vi "Initialize.vi"(8 "error in":errorcluster, 10 "parameters":variant, 11 "node in":refnum<class "control module editor.lvclass">) -> (0 "error out":errorcluster, 2 "summary":T2[](array[typedef]), 3 "data value reference":T1)   [LabVIEW 2013, in "control module editor.lvclass"]
doc: "Initializes the data of a node to its default state.\nThe object is not created inside of this VI, because it is created from a File depending on user selection."
uses:
  control module editor.lvclass
  <vilib>/NI/Configuration Framework/Node/Summary.ctl
  <vilib>/NI/Configuration Framework/Node/NodeRef.ctl
  <vilib>/NI/Configuration Framework/Node/NISE_CEF_Node.lvclass
  Configuration Editor/Classes/Module editor node/module editor node.lvclass
  configuration/control module configuration.lvclass
  read fixed channel configuration.vi
  <vilib>/NI/Configuration Framework/NISE_CEF_TreeControl.lvlib
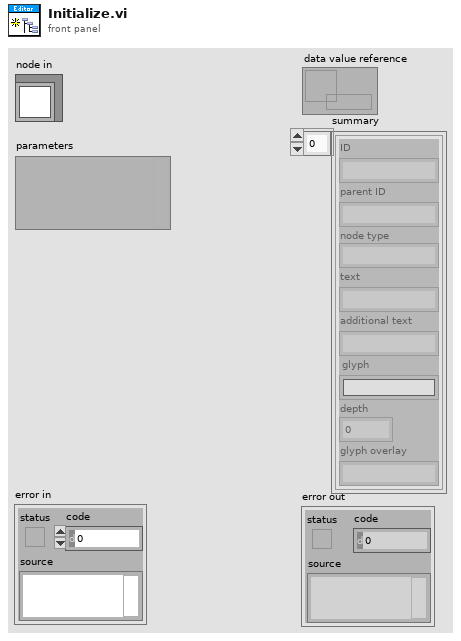
[diagram p1: front panel]
types:
  T1 = typedef "NISE_CEF_Node.lvclass/NodeRef.ctl" = refnum<data-value>
  T2 = typedef "NISE_CEF_Node.lvclass/Summary.ctl" = cluster{"ID":string, "parent ID":string, "node type":string, "text":string, "additional text":string, "glyph":string, "depth":i32, "glyph overlay":string}
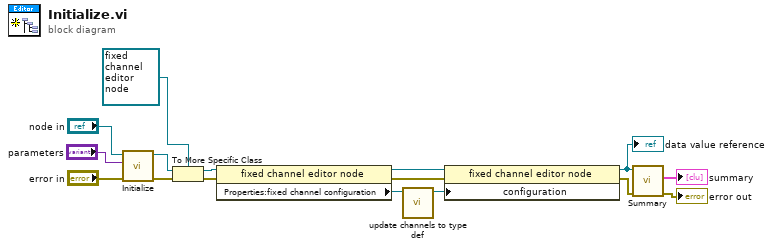
[diagram p0: block diagram]
diagram:
  n1 = call-parent "Initialize.vi"("error in"="error in", "parameters"="parameters", "node in"="node in") -> ("error out"=w16:errorcluster, "data value reference"=w12:T1)  [unwired: 6 in, 1 out]
  n2 = To More Specific Class(target class=refnum<data-value> refnum, reference=w12, error in=w16) -> (specific class reference=w6:refnum<data-value>, error out=w10:errorcluster)
  n3 = property class="fixed channel editor node"(reference=w6, error in=w10) -> (reference out=w4:refnum<data-value>, error out=w7:errorcluster, "Properties:fixed channel configuration"=w2:refnum<class "control module configuration.lvclass">)
  n4 = call-dynamic "update channels to type def.vi"("fixed channel configuration in"=w2) -> ("fixed channel configuration out"=w1:refnum<class "control module configuration.lvclass">)  [unwired: 10 in]
  n5 = property class="fixed channel editor node"(reference=w4, error in=w7, "configuration"=w1) -> (reference out=w3:refnum<data-value>, error out=w5:errorcluster)
  "data value reference" <- w3
  n6 = call <vilib>:"Summary.vi"("error in"=w5, "node self ref"=w3) -> ("error out"=→"error out":errorcluster, "summary"=→"summary":T2[])  [unwired: 8 in]
